vi "Create Class Instance.vi"() -> (3 "SimpleArithmetic.lvclass":refnum<class "SimpleArithmetic.lvclass">)   [LabVIEW 2010]
uses:
  SimpleArithmetic.lvclass
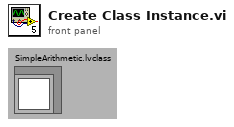
[diagram p1: front panel]
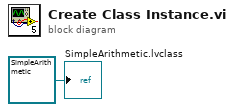
[diagram p0: block diagram]
diagram:
  "SimpleArithmetic.lvclass" <- refnum<class "SimpleArithmetic.lvclass"> refnum ("SimpleArithmetic.lvclass")
